vi "Command RPIN.vi"(0 "Serial Devices in":refnum<class "Serial Devices.lvclass">, 1 "Device":string, 7 "Port":u8, 9 "Pin":u8, 11 "error in (no error)":errorcluster) -> (4 "Serial Devices out":refnum<class "Serial Devices.lvclass">, 6 "Command":string, 10 "Expected":string, 15 "error out":errorcluster)   [LabVIEW 2019, in "Serial Devices.lvlib" / "Serial Devices.lvclass"]
uses:
  Serial Devices.lvclass
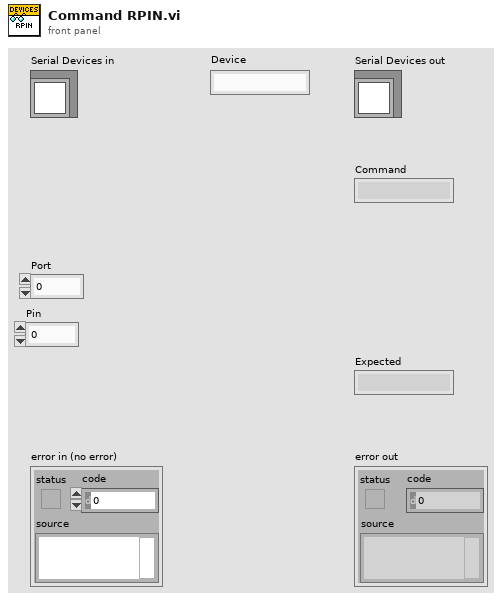
[diagram p1: front panel]
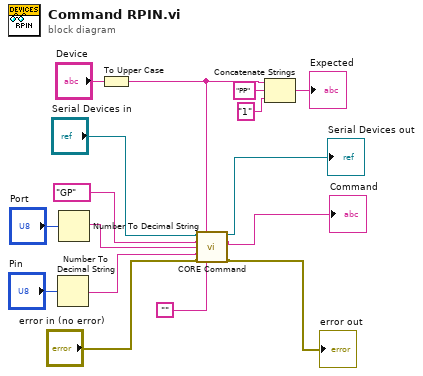
[diagram p0: block diagram]
diagram:
  n1 = Number To Decimal String(number="Pin") -> (decimal integer string=w1:string)  [unwired: 1 in]
  n2 = Number To Decimal String(number="Port") -> (decimal integer string=w9:string)  [unwired: 1 in]
  n3 = To Upper Case(1:"Device") -> (0:w6:string)
  n4 = call "CORE Command.vi"("Serial Devices in"="Serial Devices in", "Device"=w6, "Command"="GP", "Chanel-Puerto"=w9, "Param-Pin"=w1, "error in (no error)"="error in (no error)", "Valor"="") -> ("Serial Devices out"=→"Serial Devices out":refnum<class "Serial Devices.lvclass">, "Command"=→"Command":string, "error out"=→"error out":errorcluster)  [unwired: 5 in, 1 out]
  n5 = Concatenate Strings(w6, "PP" ("string"), "1" ("string")) -> (→"Expected":string)
